vi "GUID string to int.vi"(11 "uuid":string) -> (3 "GUID":T1 {"Lo" format="%.0x"; "Hi" format="%.0x"})   [LabVIEW 2023, in "CEF.lvlib" / "CEF_serializable configuration.lvclass"]
doc: "Copyright 2017 National Instruments Corporation\n\nLicensed under the Apache License, Version 2.0 (the \"License\"); you may not use this file except in compliance with the License. You may obtain a copy of the License at http://www.apache.org/licenses/LICENSE-2.0\nUnless required by applicable law or agreed to in writing, software distributed under the License is distributed on an \"AS IS\" BASIS, WITHOUT WARRANTIES OR CONDITIONS OF ANY KIND, either express or implied. See the License for the specific language governing permissions and limitations under the License."
uses:
  CEF_serializable configuration.lvclass
  Numeric GUID.ctl
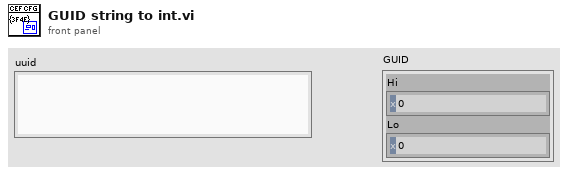
[diagram p1: front panel]
types:
  T1 = typedef "CEF.lvlib/CEF_serializable configuration.lvclass/Numeric GUID.ctl" = cluster{"Hi":u64, "Lo":u64}
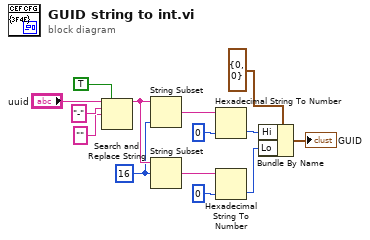
[diagram p0: block diagram]
diagram:
  w1 = 16 ("length (rest)")
  n1 = Search and Replace String(replace all?=TRUE ("replace all? (F)"), input string="uuid", search string="-" ("new element/subarray"), replace string="" ("replace string (\"\")")) -> (result string=w4:string)  [unwired: 4 in, 3 out]
  n2 = String Subset(string=w4, length (rest)=w1) -> (substring=w3:string)  [unwired: 1 in]
  n3 = String Subset(string=w4, offset (0)=w1) -> (substring=w2:string)  [unwired: 1 in]
  n4 = Hexadecimal String To Number(string=w3, default (0uL)=u64 0 ("default (0 U32)")) -> (number=w11:u64)  [unwired: 1 in, 1 out]
  n5 = Hexadecimal String To Number(string=w2, default (0uL)=u64 0 ("default (0 U32)")) -> (number=w10:u64)  [unwired: 1 in, 1 out]
  n6 = Bundle By Name(cluster=T1 {"Hi"=0, "Lo"=0} ("GUID"), "Hi"=w11, "Lo"=w10) -> (→"GUID":T1)
